vi "LINX - Seven Segment Display.vi"() -> ()   [LabVIEW 2011, in "LVH-LINX.lvlib"]
doc: "Set a seven segment LED to display a character using secven digital output channels of a LINX device."
uses:
  vi.lib/LabVIEW Hacker/LINX/LVH-LINX.lvlib
  vi.lib/LabVIEW Hacker/LINX/Private/Type Defs/Seven Segment Control.ctl
panel:
  out "Seven Seg Indicator":T1
  in  "Character":string="s"
  in  "Serial Port":refnum<visa-resource-name>
  in  "Stop Button":bool
  out "Loop Rate (Hz)":u32
  in  "DO Channels":u8[](array[numeric])
  # "Circuit Schematic"
  # "Seven Segment Output"
  # "LINX Device Settings"
  # "a"
  # "b"
  # "c"
  # "d"
  # "e"
  # "f"
  # "g"
  # "h"
  # "Seven Segment Display Example\n\nThis example demonstrates how write a character to a seven segment display using \ndigital output channels.\n\nNote: This example is configured to use a serial interface but can easily be modified\nto use TCP or run on myRIO.\n\nInstructions\n1. Select the COM Port associated with the LINX Device.\n2. Select the Digital Output Channels corresponding to the display segments.\n3. Click the Run Arrow.\n4. Change the output character to update the display."
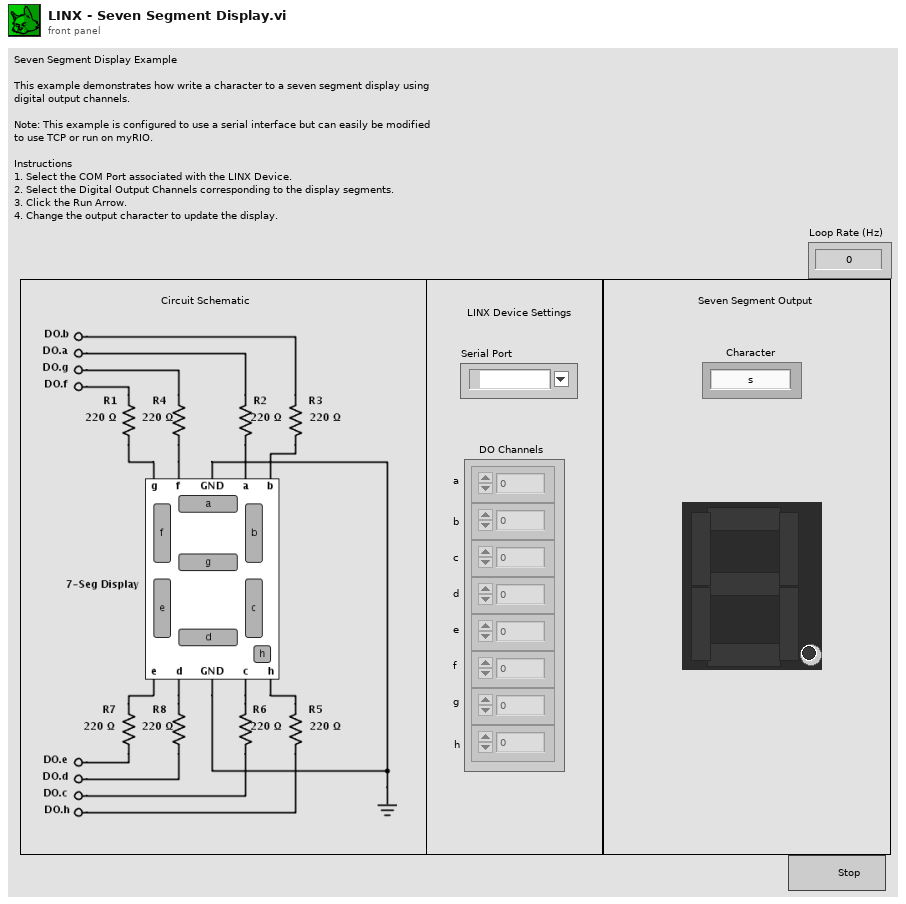
[diagram p1: front panel]
types:
  T1 = typedef "LVH-LINX.lvlib/Seven Segment Control.ctl" = cluster{"Segment 0":bool, "Segment 1":bool, "Segment 2":bool, "Segment 3":bool, "Segment 4":bool, "Segment 5":bool, "Segment 6":bool, "DP":bool}
  T2 = typedef "LVH-LINX.lvlib/LINX Ref.ctl" = cluster{"Platform":T3, "Interface":T4, "LINX Device Config":T5}
  T3 = typedef "LVH-LINX.lvlib/Platform.ctl" = enum16{"LINX", "myRIO"}
  T4 = typedef "LVH-LINX.lvlib/Interface.ctl" = enum16{"Serial", "TCP"}
  T5 = typedef "LVH-LINX.lvlib/Device.lvlib/LINX Device Config.ctl" = cluster{"Interface":T4, "COM Port":refnum<visa-resource-name>, "TCP Configuration":T6, "Device Family":u8, "Device ID":u8, "Device Name":string, "TCP Ref":refnum<k5>, "Channels":T7}
  T6 = typedef "LVH-LINX.lvlib/Device.lvlib/TCP Config.ctl" = cluster{"IP Address":string, "Port":u16}
  T7 = typedef "LVH-LINX.lvlib/Channels.ctl" = cluster{"DI":u8[], "DO":u8[], "AI":u8[], "AO":u8[], "PWM":u8[], "QE":u8[], "UART":u8[], "I2C 2":u8[], "SPI":u8[], "CAN":u8[], "Servo":u8[], "AI Ref (V)":dbl, "AO Ref (V)":dbl, "AO Resolution (Bits)":u8}
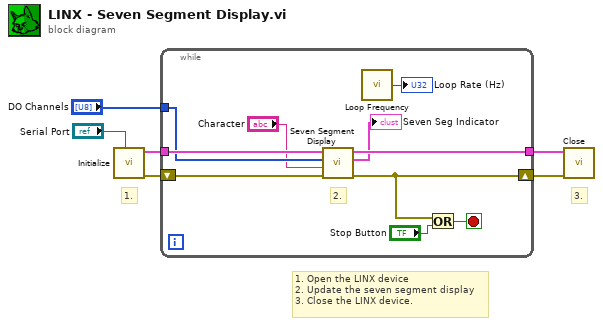
[diagram p0: block diagram]
diagram:
  # "3."
  # "1."
  # "1. Open the LINX device\n2. Update the seven segment display\n3. Close the LINX device."
  n1 = call "Initialize.vi"("Serial Port"="Serial Port") -> ("Error Out"=w2:errorcluster, "LINX Ref"=w3:T2)  [unwired: 8 in, 1 out]
  n2 = while {
    shift-right: [w11] -> w6
    shift-left: w2 -> [w10]
    tunnel: [w12] -> w4
    tunnel: w3 -> [w13]
    tunnel: "DO Channels" -> [w9]
    stop <- w16 stop-if-true
    # "2."
    n3 = call "Seven Segment Display.vi"("Error In"=w10, "Character"="Character", "Channels"=w9, "LINX Resource"=w13) -> ("Error Out"=w11:errorcluster, "Seven Seg Indicator"=→"Seven Seg Indicator":T1, "LINX Resource"=w12:T2)  [unwired: 5 in]
    n4 = call "Loop Frequency.vi"() -> ("Loop Rate (Hz)"=→"Loop Rate (Hz)":u32)
    n5 = Or(x=w11, y="Stop Button") -> (x .or. y?=w16:bool)
  }
  n6 = call "Close.vi"("Error In"=w6, "LINX Resource"=w4) -> ()  [unwired: 8 in, 2 out]
